vi "HOST_nonmixingHFoutput_3-22-23.vi"() -> ()   [LabVIEW 2020]
uses:
  <vilib>/userDefined/Silver/nirio_resource_slv.ctl
  Controls/Clock Select.ctl
  <vilib>/FPGAPlugInAG/PXIe-7972R/niLvFpga_Open_PXIe-7972R.vi
  <vilib>/rvi/interface/common/dynamic/niFpgaDynamicAddResources.vi
  <vilib>/rvi/interface/common/niFpgaWaitOnOcc.vi
  <vilib>/Utility/error.llb/Error Cluster From Error Code.vi
  <vilib>/Utility/file.llb/Write Delimited Spreadsheet (string).vi
  <vilib>/rvi/errors/niLvFpgaAdjustHostInterfaceError.vi
  <instrlib>/_niInstr/Streaming/v1/Host/Public/Start Finite Stream.vi
  <instrlib>/_niInstr/Streaming/v1/Host/Public/Wait for Stream.vi
  <instrlib>/_niInstr/Streaming/v1/Host/Public/Start Continuous Stream.vi
  <vilib>/FPGAPlugInAG/Dynamic/niLvFpga_Close_Dynamic.vi
  <vilib>/rvi/interface/nirviOpenFPGA/nirviOpenFPGA.xnode
  FPGA Bitfiles/rfsignal_FPGATarget_nonmixinghighfre_8EThLoI8BTc.lvbitx
  <vilib>/rvi/interface/nirviMethod/nirviMethod.xnode
  <vilib>/rvi/interface/nirviReadWriteControl/nirviReadWriteControl.xnode
  <vilib>/rvi/interface/nirviCloseFPGA/nirviCloseFPGA.xnode
  <vilib>/rvi/errors/niLvFpgaMergeErrorWithErrorCode.vi
  <vilib>/rvi/interface/Simulation/niFpgaSimulationCallBeginRW.vi
  <instrlib>/_niInstr/Streaming/v1/Host/niInstr Streaming v1 Host.lvlib
  NiFpgaLv.dll
  <vilib>/FPGAPlugInAG/Dynamic/niLvFpga_ReadFifo_Dynamic.vi
  <vilib>/FPGAPlugInAG/Dynamic/niLvFpga_WriteFifo_Dynamic.vi
  <vilib>/FPGAPlugInAG/Dynamic/niLvFpga_StartFifo_Dynamic.vi
  <vilib>/FPGAPlugInAG/Dynamic/niLvFpga_ConfigureFifo_Dynamic.vi
panel:
  in  "Fq Scan Step Size":dbl=100000.0 format="%0.2p"
  in  "Record time for power sweep":bool
  in  "Channel Save Selector":bool=TRUE
  in  "save path for power calibration (dialog if empty)":path
  in  "Fq Scan Endpoint":dbl[](array[numeric])=[75000000.0, 75000000.0] format="%0.2p"
  out "time check":u16=1
  in  "Cycles per step":u16=30
  in  "write time":bool
  in  "Scan Frequencies":bool
  out "Empty Elements Remaining":u32=8960
  in  "Amplitude (V)":dbl[](array[numeric])=[0.45, 0.45, 0.12, 0.12, 0.1, 0.12, 0.12, 0.12] format="%0.2p"
  in  "Frequencies (Hz)":dbl[](array[numeric])=[75000000.0, 75000000.0] format="%0.2p"
  in  "Trigger Type":enum8{"Immediate", "Data Trigger", "TRIG input"}(ring)
  in  "Clock Select":T1 items=["Internal Clock", "Internal Clock w/ Ref via CLK/REF IN", "Internal Clock w/ Ref via Sync Clock", "External Clock via CLK/REF IN"]
  in  "Rate of External Sample Clock (MHz)":u16=100 min=60 max=100 step=1
  in  "Data Trigger When":enum8{"Trigger Above", "Trigger Below"}(ring)
  in  "Sampling Info":cluster{"Fs":dbl, "#s":dbl}={"Fs"=200000000.0, "#s"=8192.0} {"Fs" format="%#_6p"}
  in  "Update Waveform":bool
  in  "Signal Type":T2(ring)
  out "AO":waveform(dbl)(graph)={"t0"=timestamp(0.0024 s since 1904-01-01), "dt"=5e-09, "Y"=array[32000 elements]}
  out "AI":waveform(dbl)[](graph)=[{"t0"=timestamp(0 s since 1904-01-01), "dt"=1e-08, "Y"=array[1024 elements]}, {"t0"=timestamp(0 s since 1904-01-01), "dt"=1e-08, "Y"=array[1024 elements]}, {"t0"=timestamp(0 s since 1904-01-01), "dt"=1e-08, "Y"=array[1024 elements]}, {"t0"=timestamp(0 s since 1904-01-01), "dt"=1e-08, "Y"=array[1024 elements]}]
  out "Error Out":errorcluster
  in  "Data Trigger Level (V)":dbl
  in  "stop":bool
  in  "Record Size":u16=1024
  in  "RIO Resource":T3="RIO0"
  # "Resource Configuration"
  # "AI Configuration"
  # "Ignored when Internal Clock is selected"
  # "AI Configuration"
  # "AO 0"
  # "A0 Configuration"
  # "AO 1"
  # "Example Description: This example acquires records of analog input data and generates analog output data from the NI 5783 adapter module.\nFor the analog input, it allows the user to select an AI channel, trigger type, and record size. For the analog output, it allows the user to select AO channel, waveform signal type, frequency, amplitude, and sampling information.  This VI is compiled for all FPGA targets by default.\n\nVI Configuration:  This example uses the NI PXIe-7976R as the FPGA target by default. To use this VI with another FPGA target, take the following steps:\n1. On the block diagram of the host VI, right-click the Open FPGA VI Reference (NI PXIe-7976R) VI and select Configure Open FPGA VI Reference.\n2. Browse for a new target by clicking the Browse button in the Open Bitfile section.\n3. Select the Bitfile that matches your device. Click OK to select this VI.\n\nRunning the VI:\n1. Select a RIO Resource that corresponds to the FPGA device configured above.\n2. Select the correct coupling (AC or DC) for the Hardware to ensure correct data scaling. \n3. Configure the Analog Input by selecting the AI Channel, Record Size, and Trigger Type. If you are using the data edge trigger type, select the trigger level in volts. \n4. Configure the Analog Output by selecting the AO Channel, Signal Type, Signal Frequency, Sampling Info, and Amplitude.\n5. Click the run arrow to run the VI.\n6. If the Trigger Type is set to Software, data is immediately sent.  If the Trigger Type is set to Data Edge, a record of data is acquired when the input signal rises above the trigger level.\n7. Click the Update Waveform button to update the memory on the FPGA with the current waveform settings."
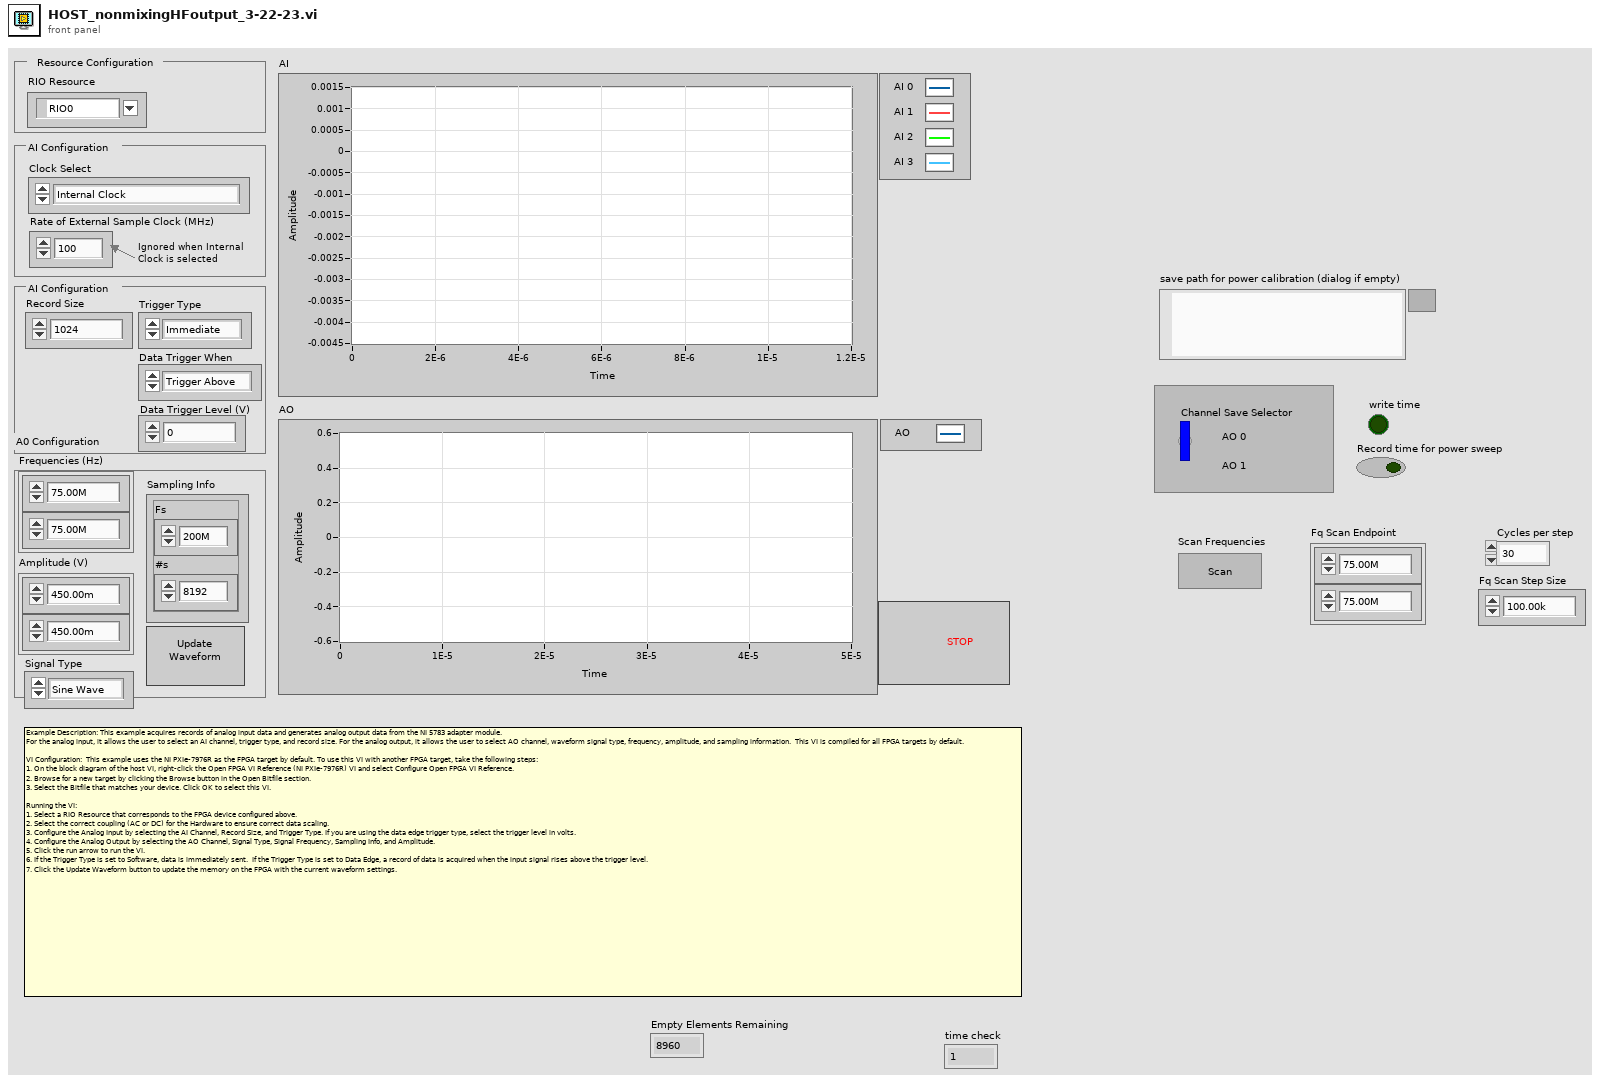
[diagram p1: front panel]
types:
  T1 = typedef "Clock Select.ctl" = u16
  T2 = enum16{"Sine Wave", "Triangle Wave", "Square Wave", "Sawtooth Wave"}
  T3 = typedef "nirio_resource_slv.ctl" = tag
  T4 = cluster{"level":i16, "trigger when":enum8{"Trigger Above", "Trigger Below"}}
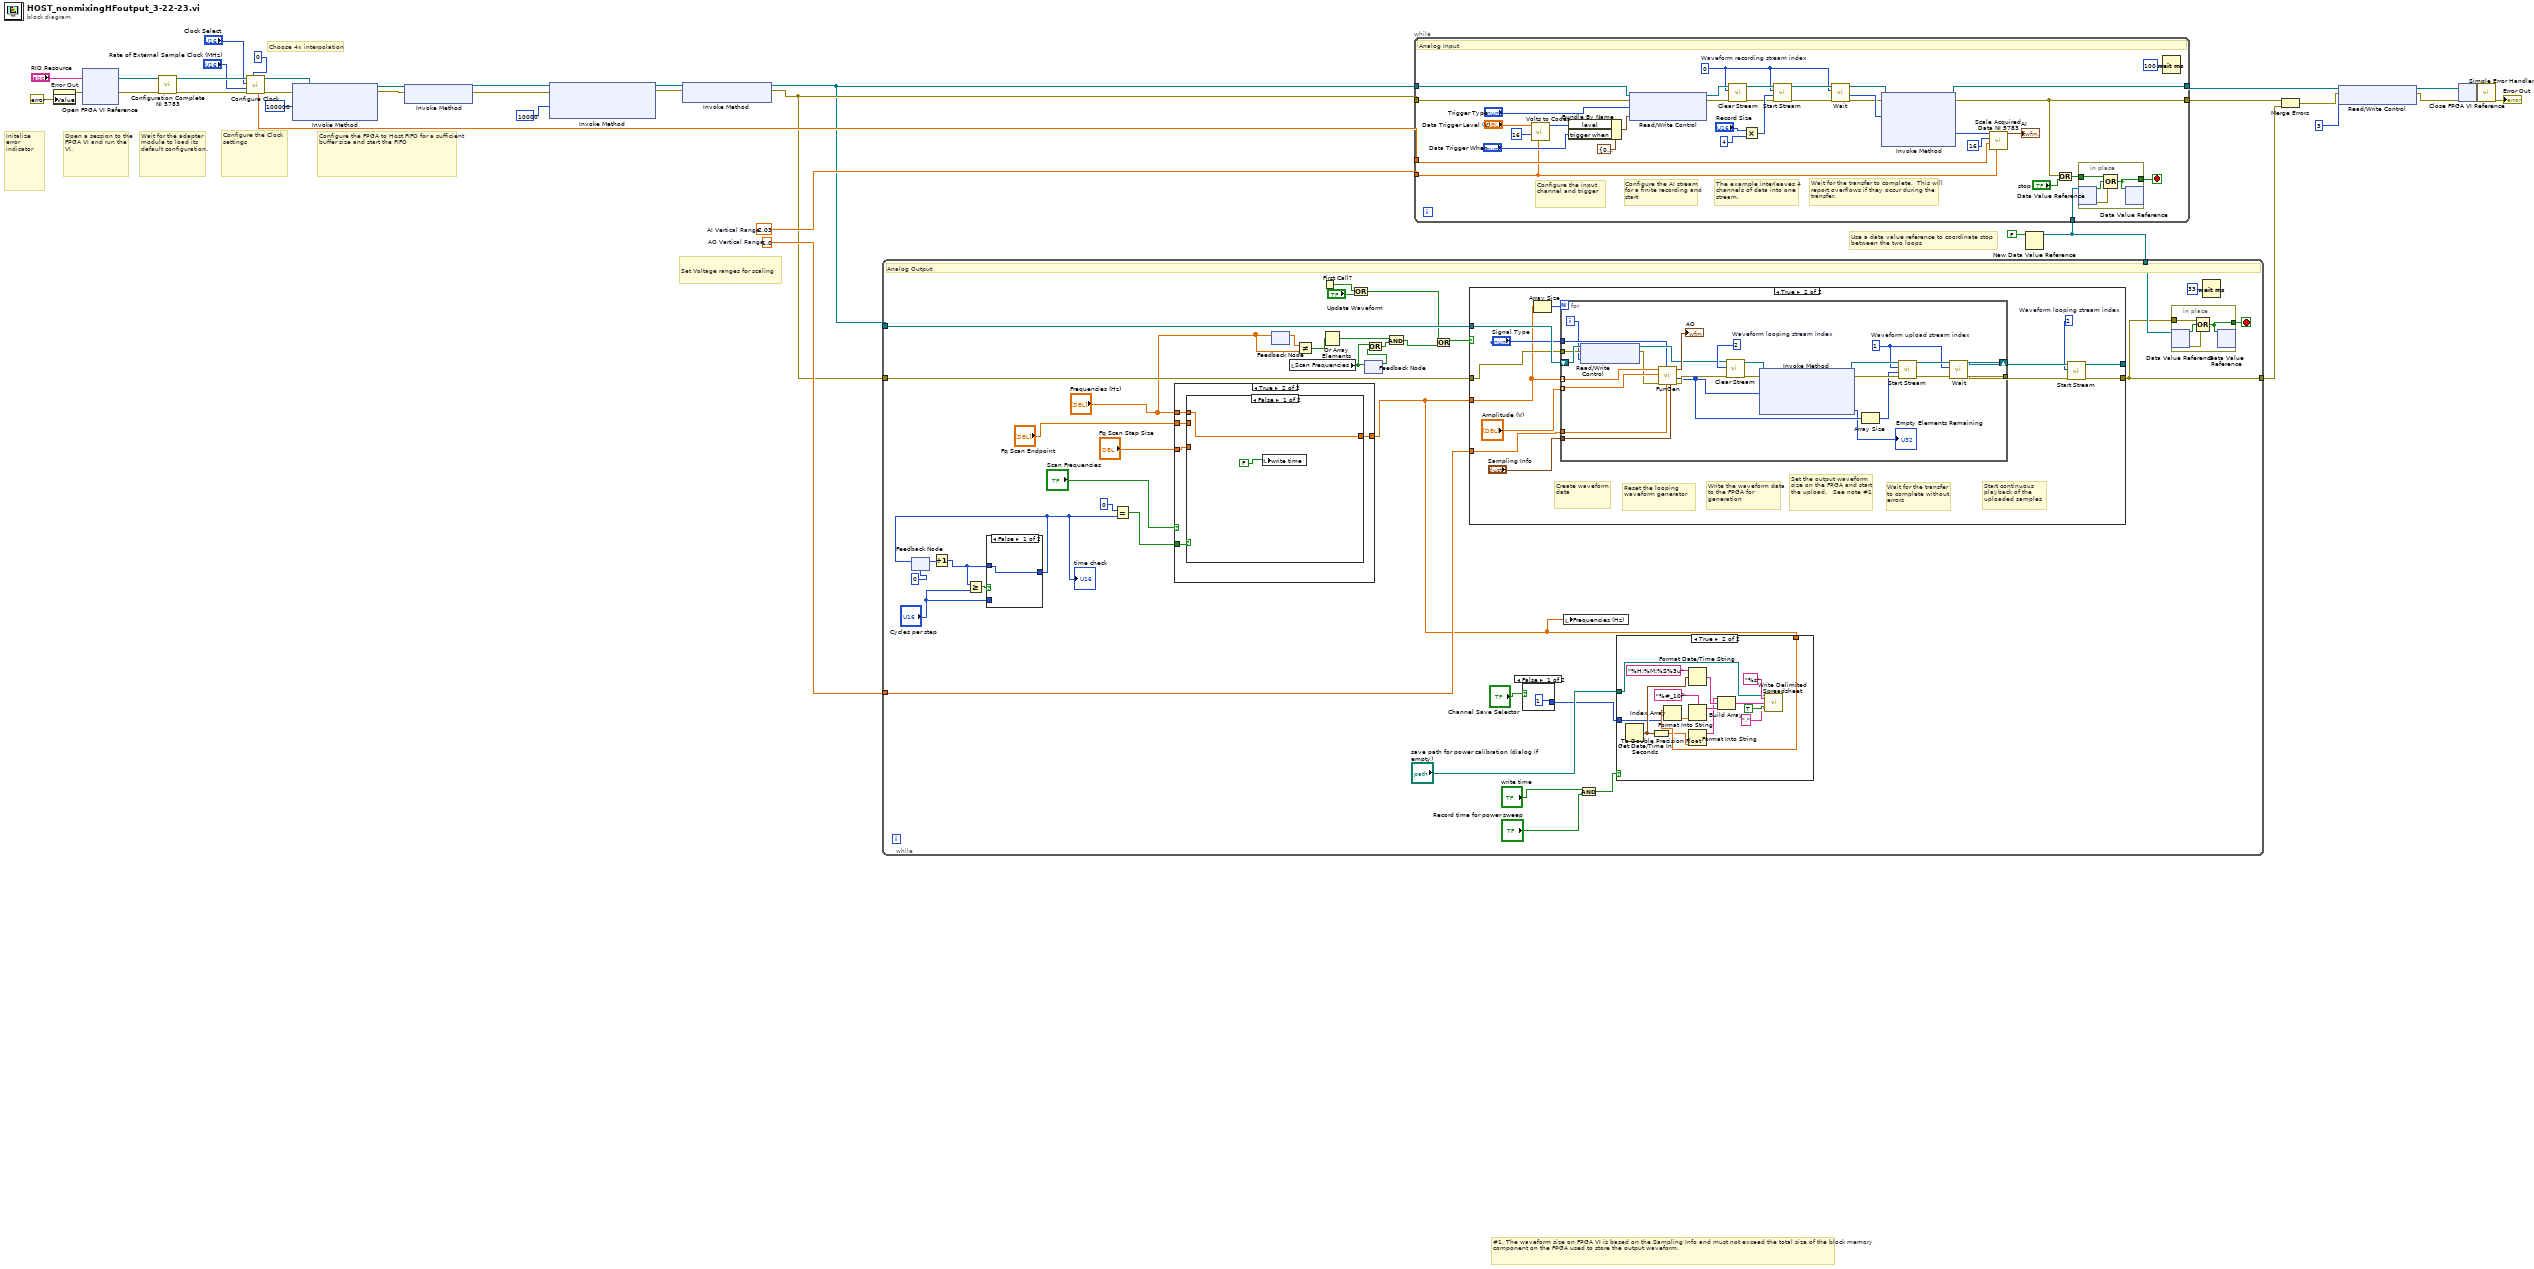
[diagram p0: block diagram]
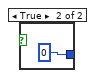
[diagram p2: hidden frame]
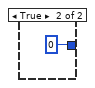
[diagram p4: hidden frame]
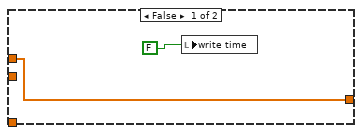
[diagram p5: hidden frame]
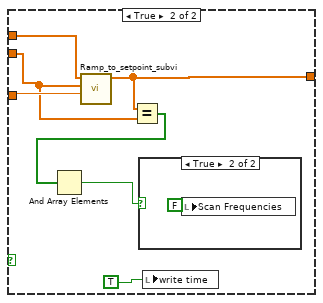
[diagram p6: hidden frame]
diagram:
  w24 = 2.03  # AI Vertical Range
  w23 = 1.0  # AO Vertical Range
  # "Choose 4x interpolation"
  # "Configure the Clock settings"
  # "Configure the FPGA to Host FIFO for a sufficient buffer size and start the FIFO"
  # "Wait for the adapter module to load its default configuration."
  # "Open a session to the FPGA VI and run the VI."
  # "Use a data value reference to coordinate stop between the two loops"
  # "Set Voltage ranges for scaling"
  # "Initalize error indicator"
  # "#1. The waveform size on FPGA VI is based on the Sampling Info and must not exceed the total size of the block memory component on the FPGA used to store the output waveform."
  n1 = property on="Error Out" class="Clust (strict)"("Value"=errorcluster {"status"=FALSE, "code"=0, "source"=""} ("error out")) -> (error out=w32:errorcluster)  [unwired: 2 in, 1 out]
  n2 = xnode "Open FPGA VI Reference"("error in"=w32, "resource name"="RIO Resource") -> ("FPGA VI Reference Out"=w22:refnum<k20>, "error out"=w21:errorcluster)
  n3 = call "Configuration Complete NI 5783.vi"("error in"=w21, "FPGA VI Reference In"=w22) -> ("error out"=w19:errorcluster, "FPGA VI Reference Out"=w20:refnum<k20>)  [unwired: 7 in, 1 out]
  n4 = call "Configure Clock.vi"("Interpolation"=0, "error in (no error)"=w19, "Rate of External Sample Clock (MHz)"="Rate of External Sample Clock (MHz)", "Clock Select"="Clock Select", "FPGA VI Reference In"=w20) -> ("error out"=w17:errorcluster, "FPGA VI Reference Out"=w18:refnum<k20>, "Sampling Rate"=w14:dbl)  [unwired: 2 in, 2 out]
  n5 = xnode "Invoke Method"("FPGA VI Reference In"=w18, "error in"=w17, "Requested Depth"=u32 100000) -> ("FPGA VI Reference Out"=w28:refnum<k20>, "error out"=w27:errorcluster)  [unwired: 1 out]
  n6 = xnode "Invoke Method"("FPGA VI Reference In"=w28, "error in"=w27) -> ("FPGA VI Reference Out"=w2:refnum<k20>, "error out"=w7:errorcluster)
  n7 = xnode "Invoke Method"("FPGA VI Reference In"=w2, "error in"=w7, "Requested Depth"=u32 10000) -> ("FPGA VI Reference Out"=w3:refnum<k20>, "error out"=w6:errorcluster)  [unwired: 1 out]
  n8 = xnode "Invoke Method"("FPGA VI Reference In"=w3, "error in"=w6) -> ("FPGA VI Reference Out"=w4:refnum<k20>, "error out"=w5:errorcluster)
  n9 = New Data Value Reference(data value=FALSE ("Stopped")) -> (data value reference=w29:refnum<data-value>)  [unwired: 1 in, 1 out]
  n10 = while {
    tunnel: w5 -> [w73]
    tunnel: [w64] -> w35
    tunnel: w4 -> [w72]
    tunnel: w23 -> [w69]
    tunnel: w29 -> [w68]
    stop <- w67 stop-if-true
    # "Analog Output"
    n11 = feedback #1(u16 0) -> (w60:u16)
    n12 = Increment(x=w60) -> (x+1=w58:u16)
    n13 = Greater Or Equal?(x=w58, y="Cycles per step") -> (x >= y?=w59:bool)
    n14 = case shown="False" w59 {
      tunnel: w58 -> [w91 _]
      tunnel: "Cycles per step" -> [_ _]
      tunnel: [w91 u16 0] -> w56
      frame False {
      }
      frame True {
      }
    }
    "time check" <- w56
    n15 = feedback-in #1(w56) -> ()
    n16 = Equal?(x=u16 0, y=w56) -> (x = y?=w55:bool)
    n17 = case shown="True" "Scan Frequencies" {
      tunnel: "Fq Scan Step Size" -> [_ w99]
      tunnel: "Frequencies (Hz)" -> [w94 w98]
      tunnel: "Fq Scan Endpoint" -> [_ w97]
      tunnel: [w94 w96] -> w47
      tunnel: w55 -> [_ w95]
      frame False {
        n18 = local write "write time"(FALSE) -> ()
      }
      frame True {
        n19 = case shown="False" w95 {
          tunnel: w98 -> [w101 w108]
          tunnel: w97 -> [_ w106]
          tunnel: w99 -> [_ w107]
          tunnel: [w101 w105] -> w96
          frame False {
            n20 = local write "write time"(FALSE) -> ()
          }
          frame True {
            n21 = call "Ramp_to_setpoint_subvi.vi"("Numeric"=w107, "Scan to Fq (CH0)"=w106, "Wave Reader CH 0 (Y)"=w108) -> ("Array"=w105:dbl[])  [unwired: 8 in]
            n22 = Equal?(x=w105, y=w106) -> (x = y?=w104:bool[])
            n23 = And Array Elements(Boolean array=w104) -> (logical AND=w102:bool)
            n24 = case shown="True" w102 {
              frame False {
              }
              frame True {
                n25 = local write "Scan Frequencies"(FALSE) -> ()
              }
            }
            n26 = local write "write time"(TRUE) -> ()
          }
        }
      }
    }
    n27 = feedback-in #2("Frequencies (Hz)") -> ()
    n28 = feedback #2() -> (w46:dbl[])  [unwired: 1 in]
    n29 = local read "Scan Frequencies"() -> (w38:bool)
    n30 = Not Equal?(x=w46, y="Frequencies (Hz)") -> (x != y?=w44:bool[])
    n31 = First Call?() -> (First Call?: T/F=w65:bool)
    n32 = Or Array Elements(Boolean array=w44) -> (logical OR=w41:bool)
    n33 = Or(x=w65, y="Update Waveform") -> (x .or. y?=w66:bool)
    n34 = feedback #3() -> (w37:bool)  [unwired: 1 in]
    n35 = feedback-in #3(w38) -> ()
    n36 = Or(x=w38, y=w37) -> (x .or. y?=w39:bool)
    n37 = And(x=w41, y=w39) -> (x .and. y?=w42:bool)
    n38 = Or(x=w66, y=w42) -> (x .or. y?=w43:bool)
    n39 = case shown="True" w43 {
      tunnel: w73 -> [w114 w120]
      tunnel: [w115 w128] -> _
      tunnel: [w114 w127] -> w64
      tunnel: w72 -> [w115 w124]
      tunnel: w69 -> [_ w118]
      tunnel: w47 -> [_ w116]
      frame False {
      }
      frame True {
        w123 = 2  # Waveform looping stream index
        # "Reset the looping waveform generator"
        # "Start continuous playback of the uploaded samples"
        # "Wait for the transfer to complete without errors"
        # "Set the output waveform size on the FPGA and start the upload.   See note #1"
        # "Write the waveform data to the FPGA for generation"
        # "Create waveform data"
        n40 = Array Size(array=w116) -> (size(s)=w122:i32)
        n41 = for {
          N: w122 -> [_]
          tunnel: [w147] -> w125
          shift-right: [w148] -> w126
          shift-left: w124 -> [w136]
          tunnel: w116 -> [w139] mode=indexing
          tunnel: "Amplitude (V)" -> [w138] mode=indexing
          tunnel: w120 -> [w135]
          tunnel: "Sampling Info" -> [w133]
          tunnel: w118 -> [w132]
          tunnel: "Signal Type" -> [w131]
          i -> [w130]
          w144 = 2  # Waveform looping stream index
          w146 = 1  # Waveform upload stream index
          n42 = xnode "Read/Write Control"("FPGA VI Reference In"=w136, "error in"=w135, "Upload selector"=w130) -> ("FPGA VI Reference Out"=w137:refnum<k20>, "error out"=w134:errorcluster)
          n43 = call "FunGen.vi"("sampling info"=w133, "range (Vpp)"=w132, "signal type"=w131, "error in (no error)"=w134, "amplitude"=w138, "frequency"=w139) -> ("error out"=w141:errorcluster, "Waveform Data"=w140:i16[], "Output Waveform (V)"=→"AO":waveform(dbl))  [unwired: 2 in, 1 out]
          n44 = call <instrlib>:"Clear Stream.vi"("error in (no error)"=w141, "stream index"=w144, "refnum in"=w137) -> ("error out"=w143:errorcluster, "refnum out"=w145:refnum<k20>)  [unwired: 7 in]
          n45 = xnode "Invoke Method"("FPGA VI Reference In"=w145, "error in"=w143, "Data"=w140) -> ("FPGA VI Reference Out"=w153:refnum<k20>, "error out"=w152:errorcluster, "Empty Elements Remaining"=→"Empty Elements Remaining":u32)  [unwired: 1 in]
          n46 = Array Size(array=w140) -> (size(s)=w151:i32)
          n47 = call-poly <instrlib>:"Start Stream.vi"("error in (no error)"=w152, "num samples"=w151, "stream index"=w146, "refnum in"=w153) -> ("error out"=w149:errorcluster, "refnum out"=w150:refnum<k20>)  [unwired: 6 in]
          n48 = call-poly <instrlib>:"Wait.vi"("error in (no error)"=w149, "stream index"=w146, "refnum in"=w150) -> ("error out"=w147:errorcluster, "refnum out"=w148:refnum<k20>)  [unwired: 5 in, 2 out]
        }
        n49 = call-poly <instrlib>:"Start Stream.vi"("error in (no error)"=w125, "stream index"=w123, "refnum in"=w126) -> ("error out"=w127:errorcluster, "refnum out"=w128:refnum<k20>)  [unwired: 7 in]
      }
    }
    n50 = case shown="False" "Channel Save Selector" {
      tunnel: [1 0] -> w52
      frame False {
      }
      frame True {
      }
    }
    n51 = local write "Frequencies (Hz)"(w47) -> ()
    n52 = And(x="write time", y="Record time for power sweep") -> (x .and. y?=w50:bool)
    n53 = case shown="True" w50 {
      tunnel: w47 -> [_ w83]
      tunnel: "save path for power calibration (dialog if empty)" -> [_ w77]
      tunnel: w52 -> [_ w76]
      frame False {
      }
      frame True {
        n54 = Get Date/Time In Seconds() -> (seconds since 1Jan1904=w80:timestamp)
        n55 = To Double Precision Float(number=w80) -> (double precision float=w79:dbl)
        n56 = Index Array(array=w83, index=w76) -> (element=w82:dbl)
        n57 = Format Date/Time String(time format string (%c)="%H:%M:%S%3u", seconds (now)=w80) -> (date/time string=w86:string)  [unwired: 1 in]
        n58 = Format Into String(format string="%#_10f", w82) -> (resulting string=w85:string)  [unwired: 2 in, 1 out]
        n59 = Format Into String(w79) -> (resulting string=w78:string)  [unwired: 3 in, 1 out]
        n60 = Build Array(w78, w86, w85) -> (w81:string[])
        n61 = call-poly <vilib>:"Write Delimited Spreadsheet.vi"("file path (dialog if empty)"=w77, "format (%s)"="%s" ("format (%.3f)"), "1D data"=w81, "append to file? (new file:F)"=TRUE, "delimiter (\\t)"="," ("delimiter (\\t)")) -> ()  [unwired: 9 in, 2 out]
      }
    }
    n62 = in-place {
      in-place-border: [w111] -> w67
      in-place-border: w64 -> [w113]
      n63 = in-place-dvr #4(w68) -> (w112:bool, w110:errorcluster)
      n64 = Compound Arithmetic op=OR(w113, w112, w110) -> (w111:bool)
      n65 = in-place-dvr #4(w111) -> ()  [unwired: 2 out]
    }
    n66 = Wait (ms)(milliseconds to wait=u32 33) -> ()  [unwired: 1 out]
  }
  n67 = while {
    tunnel: [w186] -> w12
    tunnel: w4 -> [w185]
    tunnel: w24 -> [w163]
    tunnel: w29 -> [w182]
    tunnel: w5 -> [w184]
    tunnel: [w169] -> w36
    tunnel: w14 -> [w164]
    stop <- w183 stop-if-true
    w154 = 0  # Waveform recording stream index
    # "The example interleaves 4 channels of data into one stream."
    # "Wait for the transfer to complete.  This will report overflows if they occur during the transfer."
    # "Configure the AI stream for a finite recording and start"
    # "Configure the input channel and trigger"
    # "Analog Input"
    n68 = call "Volts to Codes.vi"("range (Vpp)"=w163, "Number of Bits"=i16 16, "Volts In"="Data Trigger Level (V)") -> ("ADC Codes Out"=w165:i16)  [unwired: 8 in]
    n69 = Bundle By Name(cluster=T4 {"level"=0, "trigger when"=enum."Trigger Above"} ("Trigger Configuration"), "level"=w165, "trigger when"="Data Trigger When") -> (w168:T4)
    n70 = xnode "Read/Write Control"("FPGA VI Reference In"=w185, "error in"=w184, "Trigger Type"="Trigger Type", "Trigger Configuration"=w168) -> ("FPGA VI Reference Out"=w158:refnum<k20>, "error out"=w157:errorcluster)
    n71 = call <instrlib>:"Clear Stream.vi"("error in (no error)"=w157, "stream index"=w154, "refnum in"=w158) -> ("error out"=w156:errorcluster, "refnum out"=w155:refnum<k20>)  [unwired: 7 in]
    n72 = Multiply(x="Record Size", y=u16 4) -> (x*y=w160:u16)
    n73 = call-poly <instrlib>:"Start Stream.vi"("error in (no error)"=w156, "num samples"=w160, "stream index"=w154, "refnum in"=w155) -> ("error out"=w174:errorcluster, "refnum out"=w172:refnum<k20>)  [unwired: 6 in]
    n74 = call-poly <instrlib>:"Wait.vi"("error in (no error)"=w174, "stream index"=w154, "refnum in"=w172) -> ("error out"=w170:errorcluster, "samples transferred"=w173:u64, "refnum out"=w171:refnum<k20>)  [unwired: 5 in, 1 out]
    n75 = xnode "Invoke Method"("FPGA VI Reference In"=w171, "error in"=w170, "Number of Elements"=w173) -> ("FPGA VI Reference Out"=w186:refnum<k20>, "error out"=w169:errorcluster, "Data"=w177:i16[])  [unwired: 1 in, 1 out]
    n76 = call "Scale Acquired Data NI 5783.vi"("range (V)"=w163, "Sample Rate"=w164, "Number of Bits"=i16 16, "Data In"=w177) -> ("Data"=→"AI":waveform(dbl)[])  [unwired: 7 in]
    n77 = Or(x=w169, y="stop") -> (x .or. y?=w181:bool)
    n78 = in-place {
      in-place-border: [w189] -> w183
      in-place-border: w181 -> [w191]
      n79 = in-place-dvr #5(w182) -> (w190:bool, w188:errorcluster)
      n80 = Compound Arithmetic op=OR(w191, w190, w188) -> (w189:bool)
      n81 = in-place-dvr #5(w189) -> ()  [unwired: 2 out]
    }
    n82 = Wait (ms)(milliseconds to wait=u32 100) -> ()  [unwired: 1 out]
  }
  n83 = Merge Errors(w36, w35) -> (w10:errorcluster)
  n84 = xnode "Read/Write Control"("FPGA VI Reference In"=w12, "error in"=w10, "stream.request state 2"=3) -> ("FPGA VI Reference Out"=w11:refnum<k20>, "error out"=w9:errorcluster)
  n85 = xnode "Close FPGA VI Reference"("FPGA VI Reference In"=w11, "error in"=w9) -> ("error out"=w34:errorcluster)
  n86 = call <vilib>:"Simple Error Handler.vi"("error in (no error)"=w34) -> ("error out"=→"Error Out":errorcluster)  [unwired: 4 in, 4 out]
